vi "Set or Clear value.vi"(2 "Set clear":T3 {"target value" format="%.1p"}, 3 "Index":u32) -> ()   [LabVIEW 2019]
uses:
  TCP DAQ/Set.ctl
  TCP DAQ/clear offset.ctl
  DAQ configuration/Sensor buffer command.ctl
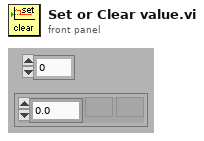
[diagram p1: front panel]
types:
  T1 = typedef "Set.ctl" = bool
  T2 = typedef "clear offset.ctl" = bool
  T3 = cluster{"Set":T1, "target value":dbl, "Clear":T2}
  T4 = typedef "Sensor buffer command.ctl" = enum16{"read average", "read recent", "read all", "write", "set buffer size", "Read channel config", "Write channel config", "clear"}
  T5 = typedef "Channel config.ctl" = cluster{"Channel Indices":T6[], "AI Max voltage":dbl[], "Calibration matrix":T7}
  T6 = typedef "channel identifier.ctl" = u16
  T7 = typedef "calib array.ctl" = T8[]
  T8 = typedef "conversion.ctl" = cluster{"conversion matrix":sgl[][], "units":string, "name":string, "scale type":T9, "offset (volts)":dbl, "second channel":i8, "correspondence table":T10, "offset (physical units)":dbl, "pH scale":T11, "D.O.":T12, "Photometer data":T13}
  T9 = typedef "scale type.ctl" = enum16{"Volts", "Polynomial", "Correspondence Table", "pH", "Dissolved Oxygen", "Quadratic", "Photometer"}
  T10 = typedef "correspondence table.ctl" = cluster{"physical units":dbl, "volts":dbl}[]
  T11 = typedef "pH scale.ctl" = cluster{"Buffers":cluster{"Buffer":dbl, "Calibrated":bool, "V/T":dbl}[], "Temperature":dbl}
  T12 = typedef "DO scale.ctl" = cluster{"Temperature":dbl, "K":dbl, "barometric pressure":dbl}
  T13 = typedef "Photometer calibration data.ctl" = cluster{"Dark Voltage":dbl, "Blank Voltage":dbl, "Standards":cluster{"Concentration":dbl, "Voltage":dbl}[]}
  T14 = typedef "Sensor data.ctl" = cluster{" Sensor array":T15[], "Time":dbl}
  T15 = typedef "sensor cluster.ctl" = cluster{"voltage":sgl, "scaled":sgl, "units":string, "Out of Range":bool}
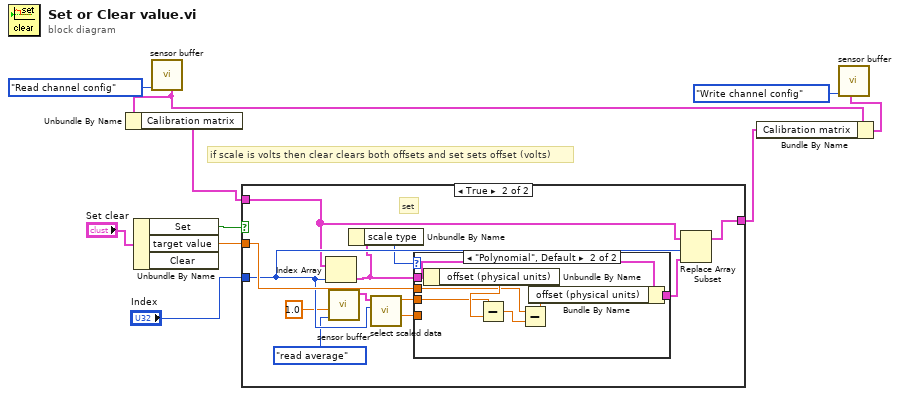
[diagram p0: block diagram]
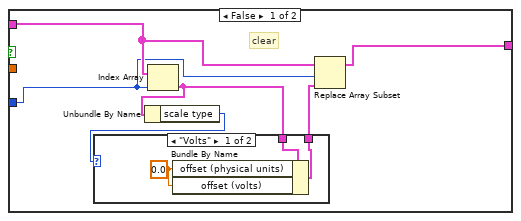
[diagram p2: hidden frame]
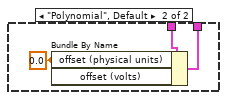
[diagram p3: hidden frame]
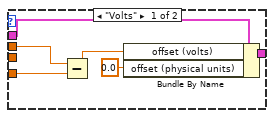
[diagram p4: hidden frame]
diagram:
  # "if scale is volts then clear clears both offsets and set sets offset (volts)"
  n1 = Unbundle By Name("Set clear") -> ("Set"=w9:T1, "target value"=w7:dbl)  [unwired: 1 out]
  n2 = call "sensor buffer.vi"("command"=Sensor_buffer_command."Read channel config") -> ("Channel Config out"=w3:T5)  [unwired: 6 in, 4 out]
  n3 = Unbundle By Name(w3) -> ("Calibration matrix"=w4:T7)
  n4 = case shown="True" w9 {
    tunnel: "Index" -> [w12 w32]
    tunnel: w4 -> [w13 w31]
    tunnel: w7 -> [_ w33]
    tunnel: [w11 w26] -> w2
    frame False {
      # "clear"
      n5 = Index Array(array=w13, index=w12) -> (element=w15:T8)
      n6 = Unbundle By Name(w15) -> ("scale type"=w16:T9)
      n7 = case shown="\"Volts\"" w16 {
        tunnel: w15 -> [w19 w22]
        tunnel: [w18 w21] -> w14
        frame "Volts" {
          w17 = 0.0 ("offset (physical units)")
          n8 = Bundle By Name(cluster=w19, "offset (physical units)"=w17, "offset (volts)"=w17) -> (w18:T8)
        }
        frame "Polynomial", Default {
          w20 = 0.0 ("offset (physical units)")
          n9 = Bundle By Name(cluster=w22, "offset (physical units)"=w20, "offset (volts)"=w20) -> (w21:T8)
        }
      }
      n10 = Replace Array Subset(array=w13, new element=w14, index=w12) -> (w11:T7)
    }
    frame True {
      # "set"
      n11 = Index Array(array=w31, index=w32) -> (element=w29:T8)
      n12 = call "sensor buffer.vi"("command"=Sensor_buffer_command."read average", "smooth interval (s)"=sgl 1.0) -> ("Calibrated data"=w25:T14)  [unwired: 5 in, 4 out]
      n13 = Unbundle By Name(w29) -> ("scale type"=w28:T9)
      n14 = call "select scaled data.vi"("Sensor index"=w32, "Sensor Data"=w25) -> ("voltage"=w27:sgl, "scaled"=w34:sgl)  [unwired: 4 in, 4 out]
      n15 = case shown="\"Polynomial\", Default" w28 {
        tunnel: w34 -> [_ w43]
        tunnel: w33 -> [w36 w42]
        tunnel: [w40 w47] -> w30
        tunnel: w29 -> [w38 w45]
        tunnel: w27 -> [w35 _]
        frame "Volts" {
          n16 = Subtract(x=w36, y=w35) -> (x-y=w39:dbl)
          n17 = Bundle By Name(cluster=w38, "offset (volts)"=w39, "offset (physical units)"=0.0) -> (w40:T8)
        }
        frame "Polynomial", Default {
          n18 = Unbundle By Name(w45) -> ("offset (physical units)"=w44:dbl)
          n19 = Subtract(x=w43, y=w44) -> (x-y=w41:dbl)
          n20 = Subtract(x=w42, y=w41) -> (x-y=w46:dbl)
          n21 = Bundle By Name(cluster=w45, "offset (physical units)"=w46) -> (w47:T8)
        }
      }
      n22 = Replace Array Subset(array=w31, new element=w30, index=w32) -> (w26:T7)
    }
  }
  n23 = Bundle By Name(cluster=w3, "Calibration matrix"=w2) -> (w1:T5)
  n24 = call "sensor buffer.vi"("Channel Config"=w1, "command"=Sensor_buffer_command."Write channel config") -> ()  [unwired: 5 in, 5 out]
